vi "Get Instrument Dependencies.vi"(8 "error in (no error)":errorcluster, 11 "Instrument in":refnum<class "Instrument.lvclass">) -> (0 "error out":errorcluster, 2 "RemoteControl out":refnum<class "RemoteControl.lvclass">, 3 "SMO out":refnum<class "Instrument.lvclass">)   [LabVIEW 2016, in "Instrument.lvclass"]
uses:
  Instrument.lvclass
  levylab_util_remote/src/RemoteControl/RemoteControl.lvclass
  C:/Program Files (x86)/National Instruments/LabVIEW 2016/vi.lib/JKI/JKI SMO/SMO/SMO.lvclass
  <vilib>/JKI/JKI SMO/SMO/SMO.lvclass
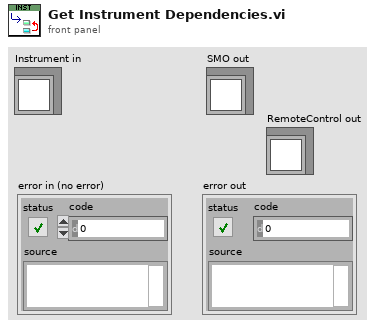
[diagram p1: front panel]
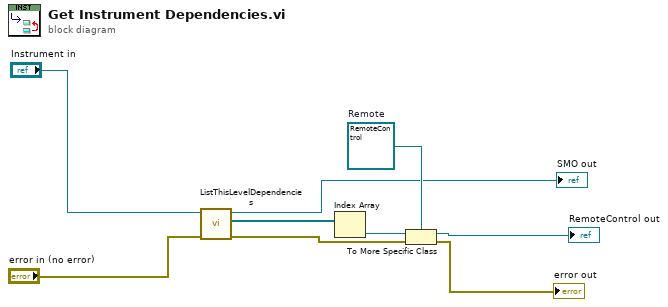
[diagram p0: block diagram]
diagram:
  w7 = refnum<class "RemoteControl.lvclass"> refnum  # Remote
  n1 = call <vilib>:"ListThisLevelDependencies.vi"("error in (no error)"="error in (no error)", "SMO in"="Instrument in") -> ("error out"=w8:errorcluster, "[My Dependencies]"=w4:refnum<class "SMO.lvclass">[], "SMO out"=→"SMO out":refnum<class "Instrument.lvclass">)  [unwired: 7 in]
  n2 = Index Array(array=w4) -> (element=w5:refnum<class "SMO.lvclass">)  [unwired: 1 in]
  n3 = To More Specific Class(target class=w7, reference=w5, error in=w8) -> (specific class reference=→"RemoteControl out":refnum<class "RemoteControl.lvclass">, error out=→"error out":errorcluster)
